vi "setUp.vi"(8 "error in (no error)":errorcluster, 11 "reference in":refnum<class "ObjectList_Delegations.lvclass">) -> (0 "error out":errorcluster, 3 "reference out":refnum<class "ObjectList_Delegations.lvclass">)   [LabVIEW 2013, in "ObjectList_Delegations.lvclass"]
doc: "setUp runs prior to the test method during test execution. Use this method to initialize any object data required by your tests."
uses:
  ObjectList_Delegations.lvclass
  <vilib>/addons/_JKI Toolkits/VI Tester/TestCase.llb/TestCase.lvclass
  Test Doubles/ListImp_RefSpy/ListImp_RefSpy.lvclass
  source/LapDog.Collections.Lists/ObjectList/ObjectList.lvclass
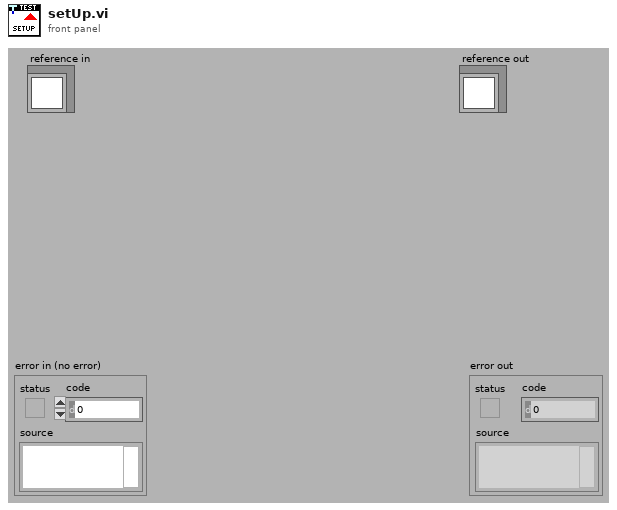
[diagram p1: front panel]
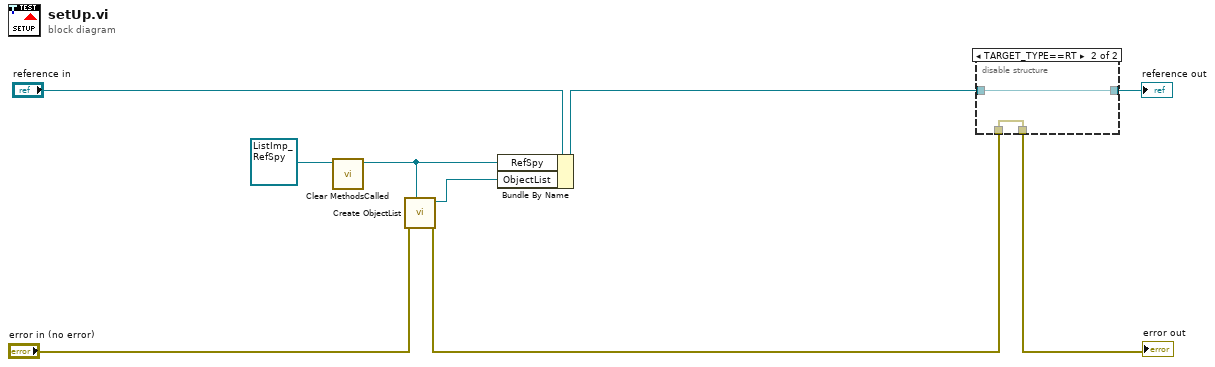
[diagram p0: block diagram]
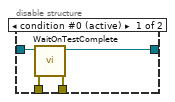
[diagram p2: hidden frame]
diagram:
  n1 = call "Clear MethodsCalled.vi"("MockListImp in"=refnum<class "ListImp_RefSpy.lvclass"> refnum ("ListImp_RefSpy.lvclass")) -> ("MockListImp out"=w4:refnum<class "ListImp_RefSpy.lvclass">)  [unwired: 9 in, 1 out]
  n2 = call "Create ObjectList.vi"("List Implementation (Array)"=w4, "error in (no error)"="error in (no error)") -> ("error out"=w1:errorcluster, "ObjectList"=w3:refnum<class "ObjectList.lvclass">)  [unwired: 8 in]
  n3 = Bundle By Name(cluster="reference in", "RefSpy"=w4, "ObjectList"=w3) -> (w6:refnum<class "ObjectList_Delegations.lvclass">)
  n4 = disable-structure shown="TARGET_TYPE==RT" {
    disable-tunnel: w1 -> [w13 w14]
    disable-tunnel: [w12 w14] -> w9
    disable-tunnel: [w11 w15] -> w7
    disable-tunnel: w6 -> [w10 w15]
    frame condition #0 (active) {
      n5 = call <vilib>:"WaitOnTestComplete.vi"("error in (no error)"=w13, "TestCase in"=w10) -> ("error out"=w12:errorcluster, "TestCase out"=w11:refnum<class "ObjectList_Delegations.lvclass">)  [unwired: 8 in]
    }
    frame condition #1 {
    }
  }
  "error out" <- w9
  "reference out" <- w7
